vi "MainEnQueue.vi"(8 "错误输入（无错误）":errorcluster, 9 "Steps":T1[](array[typedef]), 10 "CMD":enum16{"Nothing", "Insert", "Enqueue"}(ring), 11 "队列输入":refnum<queue>) -> (0 "error out":errorcluster, 3 "队列输出":refnum<queue>)   [LabVIEW 2016]
uses:
  AutoSteps.ctl
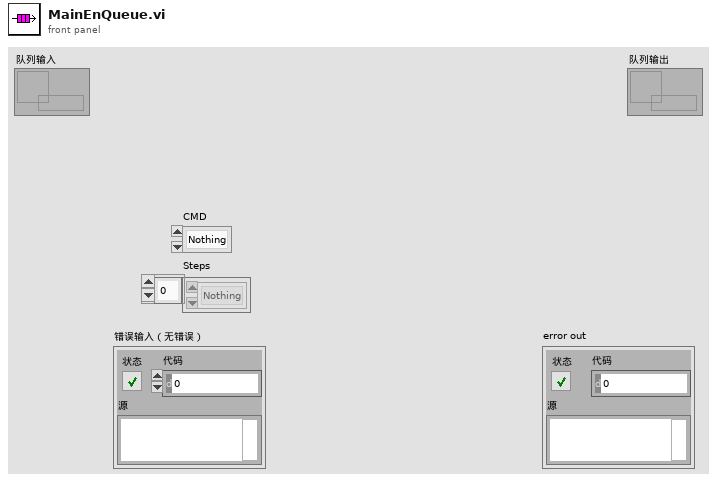
[diagram p1: front panel]
types:
  T1 = typedef "AutoSteps.ctl" = enum16{"Nothing", "Initial", "ReadConf", "Wait", "Snap", "ProcePic", "Calculate", "TrancetoPLC", "Error", "Exit"}
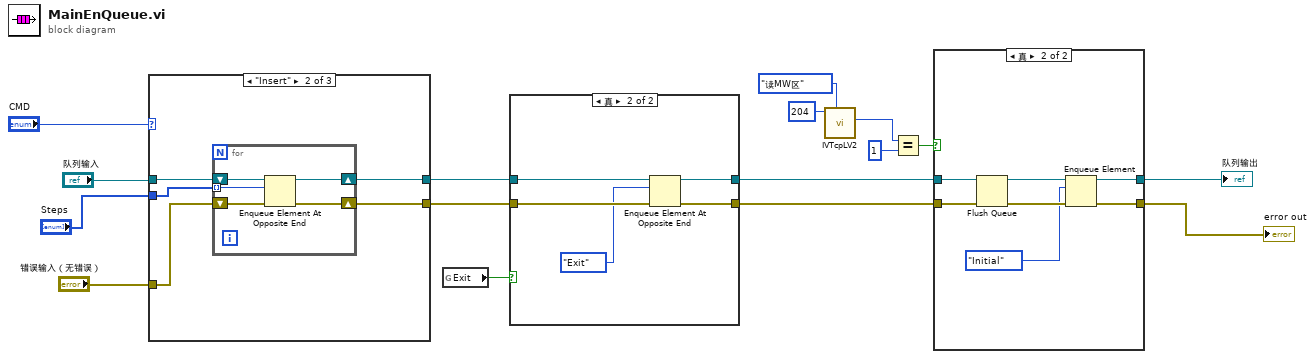
[diagram p0: block diagram]
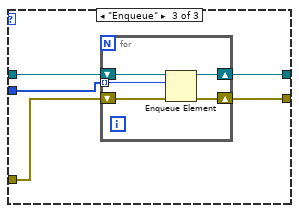
[diagram p4: hidden frame]
diagram:
  n1 = case shown="\"Insert\"" "CMD" {
    tunnel: "队列输入" -> [w18 w19 w33]
    tunnel: [w18 w23 w32] -> w15
    tunnel: [w17 w22 w31] -> w14
    tunnel: "错误输入（无错误）" -> [w17 w21 w30]
    tunnel: "Steps" -> [_ w20 w29]
    frame "Nothing", Default {
    }
    frame "Insert" {
      n2 = for {
        tunnel: w20 -> [w24] mode=indexing
        shift-right: [w27] -> w23
        shift-left: w19 -> [w28]
        shift-right: [w26] -> w22
        shift-left: w21 -> [w25]
        n3 = Enqueue Element At Opposite End(queue=w28, element=w24, error in (no error)=w25) -> (queue out=w27:refnum<queue>, error out=w26:errorcluster)  [unwired: 1 in, 1 out]
      }
    }
    frame "Enqueue" {
      n4 = for {
        tunnel: w29 -> [w34] mode=indexing
        shift-right: [w37] -> w32
        shift-left: w33 -> [w38]
        shift-right: [w36] -> w31
        shift-left: w30 -> [w35]
        n5 = Enqueue Element(queue=w38, element=w34, error in (no error)=w35) -> (queue out=w37:refnum<queue>, error out=w36:errorcluster)  [unwired: 1 in, 1 out]
      }
    }
  }
  n6 = global read "全局.vi" "Exit"() -> (w3:bool)
  n7 = case shown="真" w3 {
    tunnel: w15 -> [w40 w45]
    tunnel: [w40 w44] -> w6
    tunnel: [w39 w43] -> w5
    tunnel: w14 -> [w39 w42]
    frame False {
    }
    frame True {
      n8 = Enqueue Element At Opposite End(queue=w45, element=AutoSteps."Exit", error in (no error)=w42) -> (queue out=w44:refnum<queue>, error out=w43:errorcluster)  [unwired: 1 in, 1 out]
    }
  }
  n9 = call "IVTcpLV2.vi"("TCP操作模式"=enum16{"打开TCP", "读MW区", "写MW区", "关闭TCP"}."读MW区", "寄存器MD地址"=204) -> ("数值"=w9:u32)  [unwired: 6 in, 3 out]
  n10 = Equal?(x=w9, y=u32 1) -> (x = y?=w7:bool)
  n11 = case shown="真" w7 {
    tunnel: w6 -> [w47 w54]
    tunnel: w5 -> [w46 w53]
    tunnel: [w47 w50] -> w1
    tunnel: [w46 w49] -> w4
    frame False {
    }
    frame True {
      n12 = Flush Queue(queue=w54, error in (no error)=w53) -> (queue out=w52:refnum<queue>, error out=w51:errorcluster)  [unwired: 1 out]
      n13 = Enqueue Element(queue=w52, element=AutoSteps."Initial", error in (no error)=w51) -> (queue out=w50:refnum<queue>, error out=w49:errorcluster)  [unwired: 1 in, 1 out]
    }
  }
  "error out" <- w4
  "队列输出" <- w1
